vi "Log DSF Error.vi"(11 "error in":errorcluster) -> ()   [LabVIEW 2017, in "DSF Engine.lvlib"]
uses:
  DSF Engine.lvlib
types:
  T1 = enum16{"open", "replace", "create", "open or create", "replace or create", "replace or create with confirmation"}
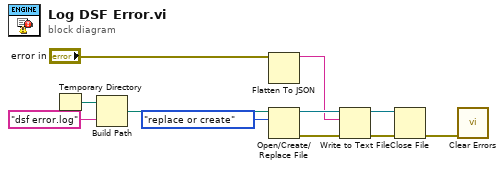
[diagram p0: block diagram]
diagram:
  n1 = Temporary Directory() -> (w6:path)
  n2 = Build Path(base path=w6, name or relative path="dsf error.log" ("file path (use dialog)")) -> (appended path=w4:path)
  n3 = Flatten To JSON(anything="error in") -> (JSON string=w2:string)  [unwired: 2 in, 1 out]
  n4 = Open/Create/Replace File(file path (use dialog)=w4, operation (0:open)=T1."replace or create") -> (refnum out=w9:refnum<file>, error out=w10:errorcluster)  [unwired: 4 in, 1 out]
  n5 = Write to Text File(file (use dialog)=w9, text=w2, error in=w10) -> (refnum out=w7:refnum<file>, error out=w8:errorcluster)  [unwired: 1 in, 1 out]
  n6 = Close File(refnum=w7, error in=w8) -> (error out=w1:errorcluster)  [unwired: 1 out]
  n7 = call <vilib>:"Clear Errors.vi"("error in (no error)"=w1) -> ()  [unwired: 5 in, 2 out]
